vi "Set Cookie.vi"(8 "error in (no error)":errorcluster, 9 "Value":string, 10 "Name":string, 11 "Response in":refnum<class "Response.lvclass">) -> (0 "error out":errorcluster, 3 "Response out":refnum<class "Response.lvclass">)   [LabVIEW 2020, in "HTTP Utils.lvlib" / "Response.lvclass"]
uses:
  Response.lvclass
  Response.lvclass/Response.ctl
  Cookie/Cookie.lvclass
  Cookie SameSite.ctl
  HTTP Utils.lvlib
  Cookie Prefix.ctl
  Cookie Attributes.ctl
panel:
  in  "Attributes (HttpOnly)":T1={"Expires"=timestamp(0 s since 1904-01-01), "Secure"=FALSE, "HttpOnly"=TRUE, "Domain"="", "Path"="", "SameSite"=enum."Unset (Lax)", "Prefix"=enum."None"}
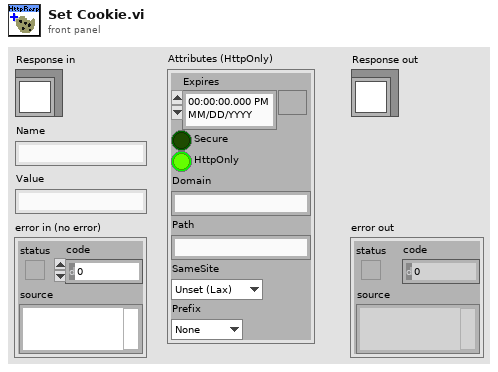
[diagram p1: front panel]
types:
  T1 = typedef "HTTP Utils.lvlib/Cookie Attributes.ctl" = cluster{"Expires":timestamp, "Secure":bool, "HttpOnly":bool, "Domain":string, "Path":string, "SameSite":T2, "Prefix":T3}
  T2 = typedef "HTTP Utils.lvlib/Cookie SameSite.ctl" = enum16{"Unset (Lax)", "Lax", "Strict", "None"}
  T3 = typedef "HTTP Utils.lvlib/Cookie Prefix.ctl" = enum16{"None", "Host", "Secure"}
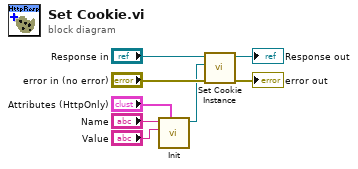
[diagram p0: block diagram]
diagram:
  n1 = call "Init.vi"("Attributes (HttpOnly)"="Attributes (HttpOnly)", "Value"="Value", "Name"="Name") -> ("Cookie out"=w3:refnum<class "Cookie.lvclass">)  [unwired: 7 in, 1 out]
  n2 = call "Set Cookie Instance.vi"("error in (no error)"="error in (no error)", "Cookie"=w3, "Response in"="Response in") -> ("error out"=→"error out":errorcluster, "Response out"=→"Response out":refnum<class "Response.lvclass">)  [unwired: 7 in]
